vi "Grouped_Proj.vi"() -> ()   [LabVIEW 2017]
uses:
  <instrlib>/Lake Shore 336/Public/Data/Sensor Data (Single Reading).vi
  <vilib>/Utility/file.llb/Write Delimited Spreadsheet (DBL).vi
  <instrlib>/Lake Shore 336/Lake Shore 336.lvlib
panel:
  in  "file to save data (dialog if empty)":path
  in  "Input (0:A)":u16(ring) items=["A", "B", "C", "D"]
  in  "Data Source (0:Kelvin)":u16(ring) items=["Kelvin", "Celsius", "Sensor Units"]
  in  "Serial Configuration":T1={"Baud Rate"=57600, "Parity"=1, "Data Bits"=7, "Stop Bits"=10, "Flow Control"=0} {"Flow Control" items=["None", "XON/XOFF", "RTS/CTS", "XON/XOFF & RTS/CTS", "DTR/DSR", "XON/XOFF & DTR/DSR"]; "Stop Bits" items=["1.0"=10, "1.5"=15, "2.0"=20]; "Data Bits" items=["7"=7, "8"=8]; "Parity" items=["None", "Odd", "Even", "Mark", "Space"]; "Baud Rate" items=["300"=300, "600"=600, "1200"=1200, "2400"=2400, "4800"=4800, "9600"=9600, "19200"=19200, "38400"=38400, "57600"=57600]}
  in  "Temperature controller name":refnum<visa-resource-name>
  in  "Resistance Range Lower Limit (2 Ohm)":dbl=2.0 format="%#_6p"
  in  "Resistance Range Upper Limit (2E+8 Ohm)":dbl=200000000.0 format="%#_6p"
  in  "Resistance NPLC (0.1)":dbl=0.1
  in  "Resistance Range (2 Ohm)":dbl=2.0
  in  "Resistance Auto Range (T: Enable)":bool=TRUE
  out "Measured Resistance (Ohms)":dbl format="%#_6p"
  out "Error Out":errorcluster
  in  "Source Meter name":refnum<visa-resource-name>="GPIB1::29::INSTR"
  in  "Error In":errorcluster
  # "Resistance vs Temperature Measurement"
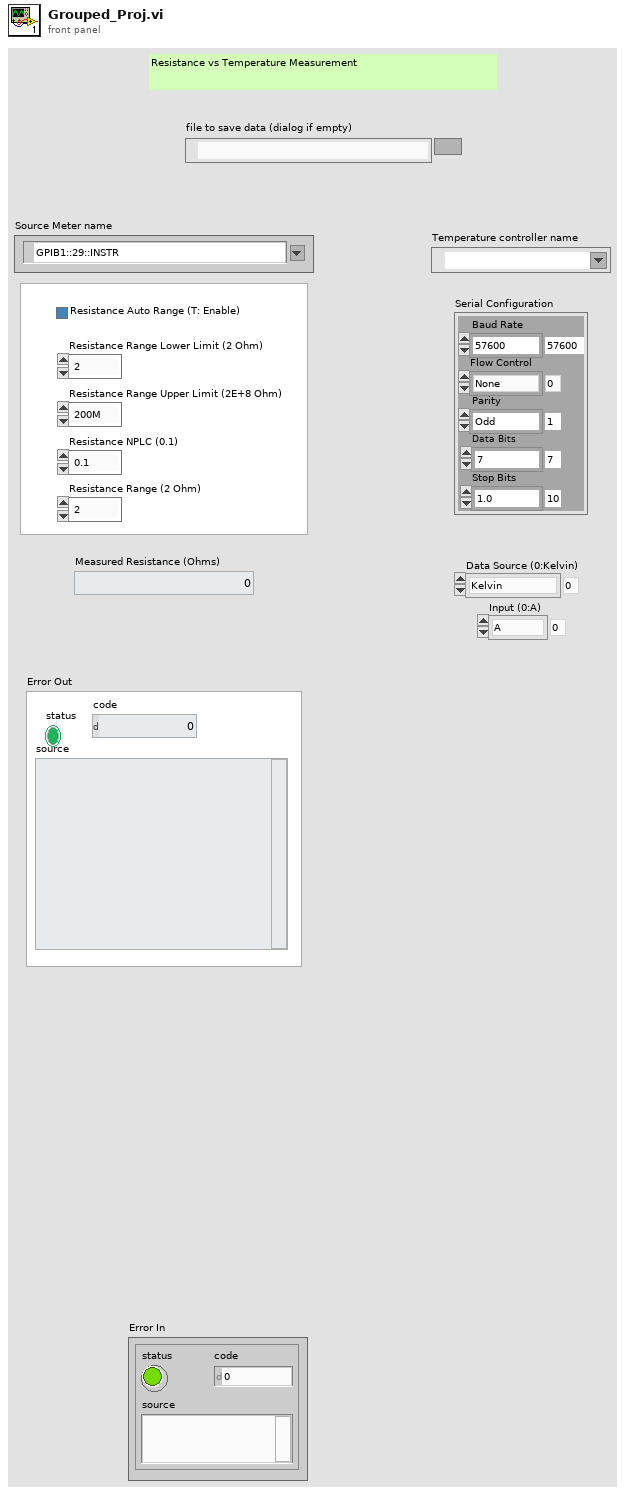
[diagram p1: front panel]
types:
  T1 = cluster{"Baud Rate":u32, "Parity":u16, "Data Bits":u16, "Stop Bits":u16, "Flow Control":u16}
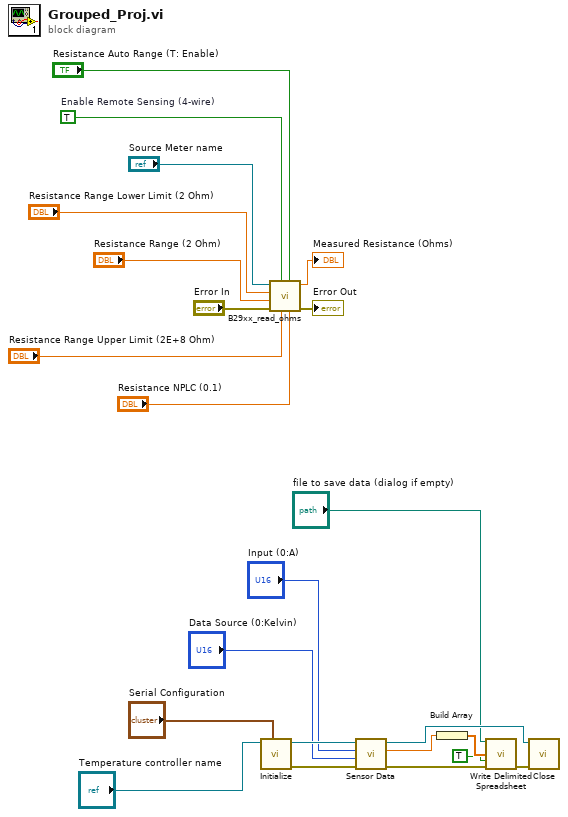
[diagram p0: block diagram]
diagram:
  w21 = TRUE  # Enable Remote Sensing (4-wire)
  n1 = call <instrlib>:"Initialize.vi"("Serial Configuration"="Serial Configuration", "VISA resource name"="Temperature controller name") -> ("error out"=w8:errorcluster, "VISA resource name out"=w11:refnum<visa-resource-name>)  [unwired: 8 in]
  n2 = call "B29xx_read_ohms.vi"("Resistance NPLC (0.1)"="Resistance NPLC (0.1)", "Resistance Auto Range (T: Enable)"="Resistance Auto Range (T: Enable)", "Resistance Range Upper Limit (2E+8 Ohm)"="Resistance Range Upper Limit (2E+8 Ohm)", "Enable Remote Sensing (4-wire)"=w21, "error in (no error)"="Error In", "Resistance Range (2 Ohm)"="Resistance Range (2 Ohm)", "Resistance Range Lower Limit (2 Ohm)"="Resistance Range Lower Limit (2 Ohm)", "VISA Refnum in"="Source Meter name") -> ("error out"=→"Error Out":errorcluster, "Measurement Result"=→"Measured Resistance (Ohms)":dbl)  [unwired: 2 in]
  n3 = call-poly <instrlib>:"Sensor Data.vi"("error in (no error)"=w8, "Data Source (0:Kelvin)"="Data Source (0:Kelvin)", "Input (0:A)"="Input (0:A)", "VISA resource name"=w11) -> ("error out"=w5:errorcluster, "Sensor Data"=w7:dbl, "VISA resource name out"=w6:refnum<visa-resource-name>)  [unwired: 5 in]
  n4 = Build Array(w7) -> (w2:dbl[])
  n5 = call-poly <vilib>:"Write Delimited Spreadsheet.vi"("file path (dialog if empty)"="file to save data (dialog if empty)", "1D data"=w2, "append to file? (new file:F)"=TRUE, "error in (no error)"=w5) -> ("error out"=w4:errorcluster)  [unwired: 10 in, 1 out]
  n6 = call <instrlib>:"Close.vi"("error in (no error)"=w4, "VISA resource name"=w6) -> ()  [unwired: 9 in, 1 out]
